vi "Status Init.vi"(8 "error in (no error)":errorcluster) -> (0 "error out":errorcluster, 3 "Status Reference":T1)   [LabVIEW 2021, in "Status.lvlib"]
uses:
  Status.lvlib
  Ctl/control.ctl
  Ctl/State.ctl
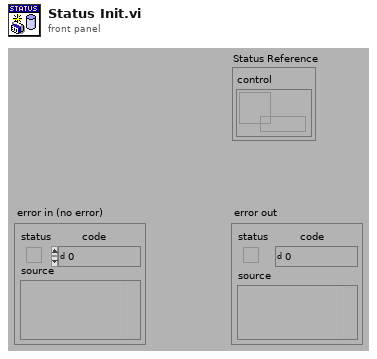
[diagram p1: front panel]
types:
  T1 = typedef "Status.lvlib/control.ctl" = cluster{"control":refnum<data-value>}
  T2 = typedef "Status.lvlib/State.ctl" = enum8{"initialization", "redefine", "standby", "connect", "wait to reconnect", "wait to reset timeout", "configure", "requests", "close connection", "stop"}
  T3 = cluster{"set_state":cluster{"Start":bool, "WrEn":bool, "Stop":bool}, "state":cluster{"errors":i32, "connect":bool, "state":T2}}
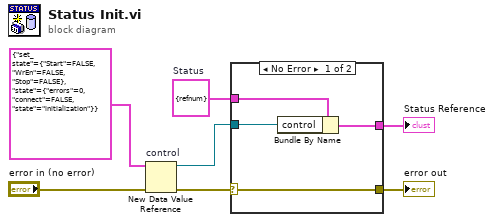
[diagram p0: block diagram]
diagram:
  w6 = T1 {"control"=refnum}  # Status
  n1 = New Data Value Reference "control"(data value=T3 {"set_state"={"Start"=FALSE, "WrEn"=FALSE, "Stop"=FALSE}, "state"={"errors"=0, "connect"=FALSE, "state"=enum."initialization"}} ("control"), error in="error in (no error)") -> (data value reference=w5:refnum<data-value>, error out=w1:errorcluster)
  n2 = case shown="No Error" w1 {
    selector: w1 -> [w9 w12]
    tunnel: w6 -> [w11 w13]
    tunnel: w5 -> [w8 _]
    tunnel: [w10 w13] -> w4
    tunnel: [w9 w12] -> w3
    frame No Error {
      n3 = Bundle By Name(cluster=w11, "control"=w8) -> (w10:T1)
    }
    frame Error {
    }
  }
  "error out" <- w3
  "Status Reference" <- w4
